vi "Test Basic Write.vi"(8 "error in (no error)":errorcluster, 11 "Scalar Channels Testing in":refnum<class "Scalar Channels Testing.lvclass">) -> (0 "error out":errorcluster, 3 "Scalar Channels Testing out":refnum<class "Scalar Channels Testing.lvclass">)   [LabVIEW 2019, in "Scalar Channels Testing.lvclass"]
uses:
  Scalar Channels Testing.lvclass
  C:/Program Files (x86)/National Instruments/LabVIEW 2019/vi.lib/NI/NI VeriStand Development Tools/NI Veristand Test Utilities/VeriStandTestCase/VeriStandTestCase.lvclass
  <vilib>/NI VeriStand/Execution/Workspace/NI VeriStand - Set Single Channel Value.vi
  <vilib>/NI VeriStand/Execution/Workspace/NI_VS Workspace ExecutionAPI.lvlib
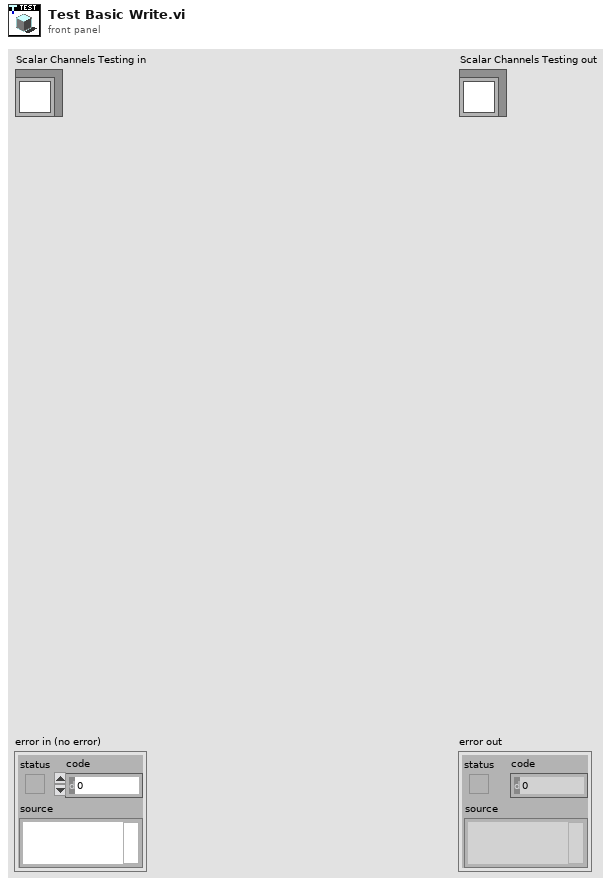
[diagram p1: front panel]
types:
  T1 = typedef "NI_VS Workspace ExecutionAPI.lvlib/WorkspaceAPI.ctl" = refnum<k24>
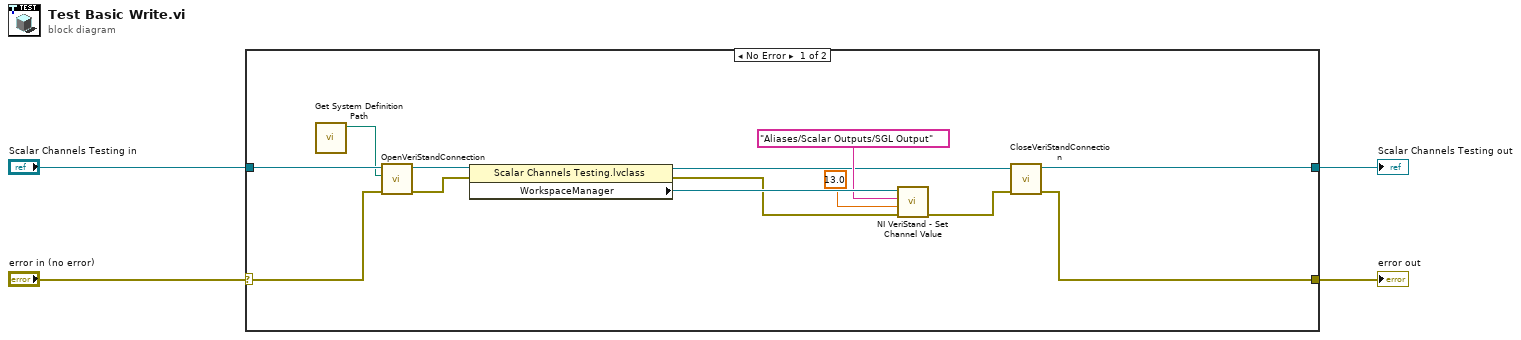
[diagram p0: block diagram]
diagram:
  n1 = case shown="No Error" "error in (no error)" {
    selector: "error in (no error)" -> [w15 w19]
    tunnel: [w14 w19] -> w3
    tunnel: [w16 w18] -> w1
    tunnel: "Scalar Channels Testing in" -> [w17 w18]
    frame No Error {
      n2 = call "Get System Definition Path.vi"() -> ("System Definition path"=w13:path)  [unwired: 11 in]
      n3 = call-dynamic "OpenVeriStandConnection.vi"("error in (no error)"=w15, "System Definition File"=w13, "VeriStand Test Case in"=w17) -> ("error out"=w11:errorcluster, "VeriStand Test Case out"=w12:refnum<class "Scalar Channels Testing.lvclass">)  [unwired: 6 in, 1 out]
      n4 = property class="Scalar Channels Testing.lvclass"(reference=w12, error in=w11) -> (reference out=w6:refnum<class "Scalar Channels Testing.lvclass">, error out=w7:errorcluster, "WorkspaceManager"=w10:T1)
      n5 = call-poly <vilib>:"NI VeriStand - Set Channel Value.vi"("error in (no error)"=w7, "Value"=13.0, "Channel"="Aliases/Scalar Outputs/SGL Output", "WorkspaceManager in"=w10) -> ("error out"=w5:errorcluster)  [unwired: 6 in, 1 out]
      n6 = call-dynamic "CloseVeriStandConnection.vi"("error in (no error)"=w5, "VeriStand Test Case in"=w6) -> ("error out"=w14:errorcluster, "VeriStand Test Case out"=w16:refnum<class "Scalar Channels Testing.lvclass">)  [unwired: 8 in]
    }
    frame Error {
    }
  }
  "error out" <- w3
  "Scalar Channels Testing out" <- w1
